vi "Configure Diode.vi"(6 "NPLC":u16(ring)=1 items=["0.0005", "1", "12", "15"], 7 "Aperture Seconds":dbl=0.016667, 8 "error in (no error)":errorcluster, 11 "VISA resource name":refnum<visa-resource-name>) -> (0 "error out":errorcluster, 3 "VISA resource name out":refnum<visa-resource-name>)   [LabVIEW 2016, in "Keithley DMM7510.lvlib"]
doc: "This VI configures the Diode measurement and the related parameters."
uses:
  Keithley DMM7510.lvlib
panel:
  in  "Bias Level":dbl=1e-05
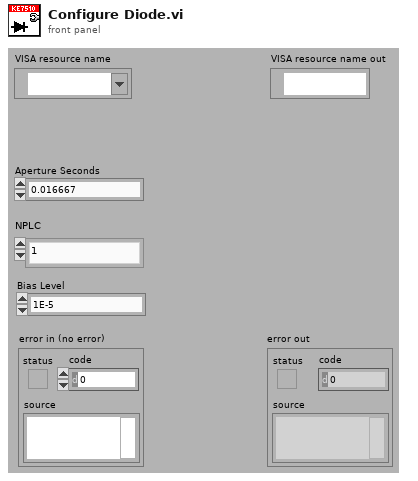
[diagram p1: front panel]
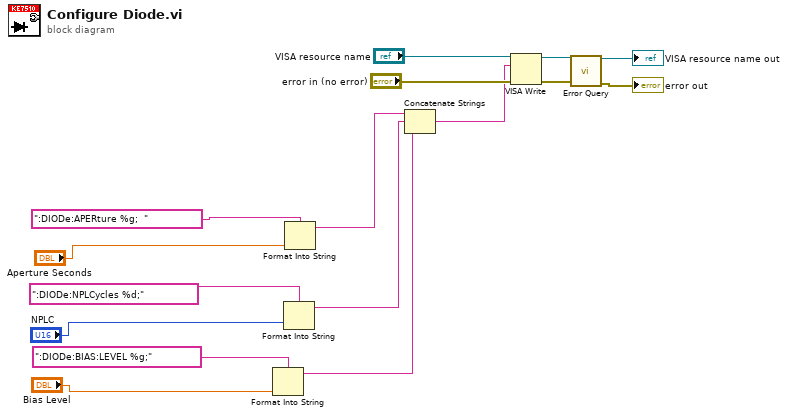
[diagram p0: block diagram]
diagram:
  n1 = Format Into String(format string=":DIODe:BIAS:LEVEL %g;", "Bias Level") -> (resulting string=w1:string)  [unwired: 2 in, 1 out]
  n2 = Format Into String(format string=":DIODe:NPLCycles %d;", "NPLC") -> (resulting string=w11:string)  [unwired: 2 in, 1 out]
  n3 = Format Into String(format string=":DIODe:APERture %g;  ", "Aperture Seconds") -> (resulting string=w12:string)  [unwired: 2 in, 1 out]
  n4 = Concatenate Strings(w12, w11, w1) -> (w10:string)
  n5 = VISA Write(VISA resource name="VISA resource name", write buffer=w10, error in (no error)="error in (no error)") -> (VISA resource name out=w9:refnum<visa-resource-name>, error out=w8:errorcluster)  [unwired: 1 out]
  n6 = call "Error Query.vi"("error in (no error)"=w8, "VISA resource name"=w9) -> ("error out"=→"error out":errorcluster, "VISA resource name out"=→"VISA resource name out":refnum<visa-resource-name>)  [unwired: 6 in, 2 out]
